vi "Func-엑셀 데이터를 그래프로 출력.vi"() -> ()   [LabVIEW 2015] (continued)
834.96\n834.98\n835\n835.01\n835.03\n835.04\n835.06\n835.08\n835.09\n835.11\n835.13\n835.14\n835.16\n835.18\n835.19\n835.21\n835.23\n835.24\n835.26\n835.28\n835.29\n835.31\n835.33\n835.34\n835.36\n835.38\n835.39\n835.41\n835.43\n835.44\n835.46\n835.48\n835.49\n835.51\n835.53\n835.54\n835.56\n835.58\n835.59\n835.61\n835.63\n835.64\n835.66\n835.68\n835.69\n835.71\n835.73\n835.74\n835.76\n835.78\n835.79\n835.81\n835.83\n835.84\n835.86\n835.88\n835.89\n835.91\n835.93\n835.94\n835.96\n835.98\n835.99\n836.01\n836.03\n836.04\n836.06\n836.08\n836.09\n836.11\n836.13\n836.14\n836.16\n836.18\n836.19\n836.21\n836.23\n836.24\n836.26\n836.28\n836.29\n836.31\n836.33\n836.34\n836.36\n836.38\n836.39\n836.41\n836.43\n836.44\n836.46\n836.48\n836.49\n836.51\n836.53\n836.54\n836.56\n836.58\n836.59\n836.61\n836.63\n836.64\n836.66\n836.68\n836.69\n836.71\n836.73\n836.74\n836.76\n836.78\n836.79\n836.81\n836.83\n836.84\n836.86\n836.88\n836.89\n836.91\n836.93\n836.94\n836.96\n836.98\n836.99\n837.01\n837.03\n837.04\n837.06\n837.08\n837.09\n837.11\n837.13\n837.14\n837.16\n837.18\n837.19\n837.21\n837.23\n837.24\n837.26\n837.28\n837.29\n837.31\n837.33\n837.34\n837.36\n837.38\n837.39\n837.41\n837.43\n837.44\n837.46\n837.48\n837.5\n837.51\n837.53\n837.54\n837.56\n837.58\n837.59\n837.61\n837.63\n837.64\n837.66\n837.68\n837.69\n837.71\n837.73\n837.75\n837.76\n837.78\n837.79\n837.81\n837.83\n837.85\n837.86\n837.88\n837.89\n837.91\n837.93\n837.94\n837.96\n837.98\n837.99\n838.01\n838.03\n838.04\n838.06\n838.08\n838.09\n838.11\n838.13\n838.14\n838.16\n838.18\n838.2\n838.21\n838.23\n838.24\n838.26\n838.28\n838.29\n838.31\n838.33\n838.34\n838.36\n838.38\n838.39\n838.41\n838.43\n838.44\n838.46\n838.48\n838.49\n838.51\n838.53\n838.54\n838.56\n838.58\n838.59\n838.61\n838.63\n838.65\n838.66\n838.68\n838.7\n838.71\n838.73\n838.74\n838.76\n838.78\n838.79\n838.81\n838.83\n838.84\n838.86\n838.88\n838.89\n838.91\n838.93\n838.94\n838.96\n838.98\n838.99\n839.01\n839.03\n839.05\n839.06\n839.08\n839.09\n839.11\n839.13\n839.14\n839.16\n839.18\n839.19\n839.21\n839.23\n839.24\n839.26\n839.28\n839.29\n839.31\n839.33\n839.34\n839.36\n839.38\n839.39\n839.41\n839.43\n839.44\n839.46\n839.48\n839.49\n839.51\n839.53\n839.54\n839.56\n839.58\n839.59\n839.61\n839.63\n839.64\n839.66\n839.68\n839.69\n839.71\n839.73\n839.74\n839.76\n839.78\n839.79\n839.81\n839.83\n839.84\n839.86\n839.88\n839.89\n839.91\n839.93\n839.94\n839.96\n839.98\n839.99\n840.01\n840.03\n840.04\n840.06\n840.08\n840.09\n840.11\n840.13\n840.15\n840.16\n840.18\n840.19\n840.21\n840.23\n840.25\n840.26\n840.28\n840.29\n840.31\n840.33\n840.34\n840.36\n840.38\n840.39\n840.41\n840.43\n840.44\n840.46\n840.48\n840.5\n840.51\n840.53\n840.54\n840.56\n840.58\n840.6\n840.61\n840.63\n840.64\n840.66\n840.68\n840.69\n840.71\n840.73\n840.74\n840.76\n840.78\n840.79\n840.81\n840.83\n840.85\n840.86\n840.88\n840.89\n840.91\n840.93\n840.95\n840.96\n840.98\n840.99\n841.01\n841.03\n841.04\n841.06\n841.08\n841.1\n841.11\n841.13\n841.14\n841.16\n841.18\n841.19\n841.21\n841.23\n841.24\n841.26\n841.28\n841.29\n841.31\n841.33\n841.34\n841.36\n841.38\n841.39\n841.41\n841.43\n841.45\n841.46\n841.48\n841.49\n841.51\n841.53\n841.54\n841.56\n841.58\n841.59\n841.61\n841.63\n841.64\n841.66\n841.68\n841.69\n841.71\n841.73\n841.74\n841.76\n841.78\n841.79\n841.81\n841.83\n841.84\n841.86\n841.88\n841.89\n841.91\n841.93\n841.94\n841.96\n841.98\n842\n842.01\n842.03\n842.04\n842.06\n842.08\n842.09\n842.11\n842.13\n842.14\n842.16\n842.18\n842.19\n842.21\n842.23\n842.24\n842.26\n842.28\n842.29\n842.31\n842.33\n842.34\n842.36\n842.38\n842.39\n842.41\n842.43\n842.44\n842.46\n842.48\n842.49\n842.51\n842.53\n842.54\n842.56\n842.58\n842.59\n842.61\n842.63\n842.64\n842.66\n842.68\n842.69\n842.71\n842.73\n842.74\n842.76\n842.78\n842.79\n842.81\n842.83\n842.84\n842.86\n842.88\n842.89\n842.91\n842.93\n842.94\n842.96\n842.98\n843\n843.01\n843.03\n843.04\n843.06\n843.08\n843.09\n843.11\n843.13\n843.14\n843.16\n843.18\n843.19\n843.21\n843.23\n843.25\n843.26\n843.28\n843.29\n843.31\n843.33\n843.34\n843.36\n843.38\n843.39\n843.41\n843.43\n843.44\n843.46\n843.48\n843.49\n843.51\n843.53\n843.54\n843.56\n843.58\n843.6\n843.61\n843.63\n843.64\n843.66\n843.68\n843.7\n843.71\n843.73\n843.74\n843.76\n843.78\n843.79\n843.81\n843.83\n843.85\n843.86\n843.88\n843.89\n843.91\n843.93\n843.95\n843.96\n843.98\n843.99\n844.01\n844.03\n844.04\n844.06\n844.08\n844.09\n844.11\n844.13\n844.14\n844.16\n844.18\n844.2\n844.21\n844.23\n844.24\n844.26\n844.28\n844.3\n844.31\n844.33\n844.34\n844.36\n844.38\n844.4\n844.41\n844.43\n844.44\n844.46\n844.48\n844.49\n844.51\n844.53\n844.55\n844.56\n844.58\n844.59\n844.61\n844.63\n844.64\n844.66\n844.68\n844.69\n844.71\n844.73\n844.74\n844.76\n844.78\n844.79\n844.81\n844.83\n844.84\n844.86\n844.88\n844.9\n844.91\n844.93\n844.94\n844.96\n844.98\n844.99\n845.01\n845.03\n845.04\n845.06\n845.08\n845.09\n845.11\n845.13\n845.14\n845.16\n845.18\n845.19\n845.21\n845.23\n845.24\n845.26\n845.28\n845.29\n845.31\n845.33\n845.34\n845.36\n845.38\n845.39\n845.41\n845.43\n845.44\n845.46\n845.48\n845.49\n845.51\n845.53\n845.54\n845.56\n845.58\n845.59\n845.61\n845.63\n845.64\n845.66\n845.68\n845.69\n845.71\n845.73\n845.74\n845.76\n845.78\n845.79\n845.81\n845.83\n845.84\n845.86\n845.88\n845.89\n845.91\n845.93\n845.94\n845.96\n845.98\n845.99\n846.01\n846.03\n846.04\n846.06\n846.08\n846.09\n846.11\n846.13\n846.14\n846.16\n846.18\n846.19\n846.21\n846.23\n846.24\n846.26\n846.28\n846.29\n846.31\n846.33\n846.35\n846.36\n846.38\n846.39\n846.41\n846.43\n846.44\n846.46\n846.48\n846.49\n846.51\n846.53\n846.54\n846.56\n846.58\n846.59\n846.61\n846.63\n846.64\n846.66\n846.68\n846.7\n846.71\n846.73\n846.74\n846.76\n846.78\n846.79\n846.81\n846.83\n846.84\n846.86\n846.88\n846.89\n846.91\n846.93\n846.95\n846.96\n846.98\n846.99\n847.01\n847.03\n847.05\n847.06\n847.08\n847.09\n847.11\n847.13\n847.14\n847.16\n847.18\n847.19\n847.21\n847.23\n847.24\n847.26\n847.28\n847.3\n847.31\n847.33\n847.34\n847.36\n847.38\n847.4\n847.41\n847.43\n847.44\n847.46\n847.48\n847.49\n847.51\n847.53\n847.55\n847.56\n847.58\n847.59\n847.61\n847.63\n847.64\n847.66\n847.68\n847.69\n847.71\n847.73\n847.75\n847.76\n847.78\n847.79\n847.81\n847.83\n847.84\n847.86\n847.88\n847.9\n847.91\n847.93\n847.94\n847.96\n847.98\n848\n848.01\n848.03\n848.04\n848.06\n848.08\n848.09\n848.11\n848.13\n848.15\n848.16\n848.18\n848.19\n848.21\n848.23\n848.24\n848.26\n848.28\n848.29\n848.31\n848.33\n848.34\n848.36\n848.38\n848.39\n848.41\n848.43\n848.44\n848.46\n848.48\n848.49\n848.51\n848.53\n848.54\n848.56\n848.58\n848.59\n848.61\n848.63\n848.64\n848.66\n848.68\n848.69\n848.71\n848.73\n848.74\n848.76\n848.78\n848.79\n848.81\n848.83\n848.84\n848.86\n848.88\n848.89\n848.91\n848.93\n848.94\n848.96\n848.98\n848.99\n849.01\n849.03\n849.04\n849.06\n849.08\n849.09\n849.11\n849.13\n849.14\n849.16\n849.18\n849.19\n849.21\n849.23\n849.24\n849.26\n849.28\n849.29\n849.31\n849.33\n849.34\n849.36\n849.38\n849.39\n849.41\n849.43\n849.45\n849.46\n849.48\n849.49\n849.51\n849.53\n849.54\n849.56\n849.58\n849.59\n849.61\n849.63\n849.64\n849.66\n849.68\n849.7\n849.71\n849.73\n849.74\n849.76\n849.78\n849.8\n849.81\n849.83\n849.84\n849.86\n849.88\n849.89\n849.91\n849.93\n849.94\n849.96\n849.98\n849.99\n850.01\n850.03\n850.05\n850.06\n850.08\n850.09\n850.11\n850.13\n850.15\n850.16\n850.18\n850.19\n850.21\n850.23\n850.24\n850.26\n850.28\n850.29\n850.31\n850.33\n850.34\n850.36\n850.38\n850.39\n850.41\n850.43\n850.44\n850.46\n850.48\n850.5\n850.51\n850.53\n850.54\n850.56\n850.58\n850.6\n850.61\n850.63\n850.64\n850.66\n850.68\n850.69\n850.71\n850.73\n850.74\n850.76\n850.78\n850.79\n850.81\n850.83\n850.85\n850.86\n850.88\n850.89\n850.91\n850.93\n850.94\n850.96\n850.98\n850.99\n851.01\n851.03\n851.04\n851.06\n851.08\n851.1\n851.11\n851.13\n851.14\n851.16\n851.18\n851.19\n851.21\n851.23\n851.24\n851.26\n851.28\n851.29\n851.31\n851.33\n851.34\n851.36\n851.38\n851.39\n851.41\n851.43\n851.44\n851.46\n851.48\n851.49\n851.51\n851.53\n851.54\n851.56\n851.58\n851.59\n851.61\n851.63\n851.64\n851.66\n851.68\n851.69\n851.71\n851.73\n851.74\n851.76\n851.78\n851.79\n851.81\n851.83\n851.84\n851.86\n851.88\n851.89\n851.91\n851.93\n851.94\n851.96\n851.98\n851.99\n852.01\n852.03\n852.04\n852.06\n852.08\n852.09\n852.11\n852.13\n852.14\n852.16\n852.18\n852.19\n852.21\n852.23\n852.24\n852.26\n852.28\n852.29\n852.31\n852.33\n852.34\n852.36\n852.38\n852.39\n852.41\n852.43\n852.44\n852.46\n852.48\n852.49\n852.51\n852.53\n852.54\n852.56\n852.58\n852.59\n852.61\n852.63\n852.64\n852.66\n852.68\n852.69\n852.71\n852.73\n852.74\n852.76\n852.78\n852.8\n852.81\n852.83\n852.84\n852.86\n852.88\n852.9\n852.91\n852.93\n852.94\n852.96\n852.98\n852.99\n853.01\n853.03\n853.04\n853.06\n853.08\n853.09\n853.11\n853.13\n853.15\n853.16\n853.18\n853.19\n853.21\n853.23\n853.25\n853.26\n853.28\n853.29\n853.31\n853.33\n853.34\n853.36\n853.38\n853.39\n853.41\n853.43\n853.44\n853.46\n853.48\n853.5\n853.51\n853.53\n853.54\n853.56\n853.58\n853.59\n853.61\n853.63\n853.64\n853.66\n853.68\n853.7\n853.71\n853.73\n853.74\n853.76\n853.78\n853.79\n853.81\n853.83\n853.84\n853.86\n853.88\n853.89\n853.91\n853.93\n853.94\n853.96\n853.98\n853.99\n854.01\n854.03\n854.04\n854.06\n854.08\n854.1\n854.11\n854.13\n854.14\n854.16\n854.18\n854.2\n854.21\n854.23\n854.24\n854.26\n854.28\n854.29\n854.31\n854.33\n854.34\n854.36\n854.38\n854.39\n854.41\n854.43\n854.44\n854.46\n854.48\n854.49\n854.51\n854.53\n854.54\n854.56\n854.58\n854.59\n854.61\n854.63\n854.64\n854.66\n854.68\n854.69\n854.71\n854.73\n854.74\n854.76\n854.78\n854.79\n854.81\n854.83\n854.84\n854.86\n854.88\n854.89\n854.91\n854.93\n854.94\n854.96\n854.98\n854.99\n855.01\n855.03\n855.04\n855.06\n855.08\n855.09\n855.11\n855.13\n855.14\n855.16\n855.18\n855.19\n855.21\n855.23\n855.24\n855.26\n855.28\n855.29\n855.31\n855.33\n855.34\n855.36\n855.38\n855.39\n855.41\n855.43\n855.44\n855.46\n855.48\n855.49\n855.51\n855.53\n855.55\n855.56\n855.58\n855.59\n855.61\n855.63\n855.64\n855.66\n855.68\n855.69\n855.71\n855.73\n855.74\n855.76\n855.78\n855.79\n855.81\n855.83\n855.84\n855.86\n855.88\n855.9\n855.91\n855.93\n855.94\n855.96\n855.98\n856\n856.01\n856.03\n856.04\n856.06\n856.08\n856.09\n856.11\n856.13\n856.15\n856.16\n856.18\n856.19\n856.21\n856.23\n856.25\n856.26\n856.28\n856.29\n856.31\n856.33\n856.35\n856.36\n856.38\n856.39\n856.41\n856.43\n856.44\n856.46\n856.48\n856.49\n856.51\n856.53\n856.54\n856.56\n856.58\n856.6\n856.61\n856.63\n856.64\n856.66\n856.68\n856.69\n856.71\n856.73\n856.74\n856.76\n856.78\n856.79\n856.81\n856.83\n856.84\n856.86\n856.88\n856.89\n856.91\n856.93\n856.94\n856.96\n856.98\n856.99\n857.01\n857.03\n857.05\n857.06\n857.08\n857.1\n857.11\n857.13\n857.14\n857.16\n857.18\n857.19\n857.21\n857.23\n857.24\n857.26\n857.28\n857.3\n857.31\n857.33\n857.34\n857.36\n857.38\n857.39\n857.41\n857.43\n857.44\n857.46\n857.48\n857.49\n857.51\n857.53\n857.54\n857.56\n857.58\n857.59\n857.61\n857.63\n857.64\n857.66\n857.68\n857.69\n857.71\n857.73\n857.74\n857.76\n857.78\n857.79\n857.81\n857.83\n857.84\n857.86\n857.88\n857.89\n857.91\n857.93\n857.94\n857.96\n857.98\n857.99\n858.01\n858.03\n858.04\n858.06\n858.08\n858.09\n858.11\n858.13\n858.14\n858.16\n858.18\n858.19\n858.21\n858.23\n858.24\n858.26\n858.28\n858.29\n858.31\n858.33\n858.34\n858.36\n858.38\n858.39\n858.41\n858.43\n858.44\n858.46\n858.48\n858.49\n858.51\n858.53\n858.54\n858.56\n858.58\n858.59\n858.61\n858.63\n858.64\n858.66\n858.68\n858.69\n858.71\n858.73\n858.74\n858.76\n858.78\n858.79\n858.81\n858.83\n858.84\n858.86\n858.88\n858.89\n858.91\n858.93\n858.94\n858.96\n858.98\n859\n859.01\n859.03\n859.04\n859.06\n859.08\n859.09\n859.11\n859.13\n859.14\n859.16\n859.18\n859.19\n859.21\n859.23\n859.25\n859.26\n859.28\n859.29\n859.31\n859.33\n859.35\n859.36\n859.38\n859.39\n859.41\n859.43\n859.45\n859.46\n859.48\n859.49\n859.51\n859.53\n859.54\n859.56\n859.58\n859.59\n859.61\n859.63\n859.64\n859.66\n859.68\n859.69\n859.71\n859.73\n859.74\n859.76\n859.78\n859.79\n859.81\n859.83\n859.84\n859.86\n859.88\n859.89\n859.91\n859.93\n859.94\n859.96\n859.98\n859.99\n860.01\n860.03\n860.04\n860.06\n860.08\n860.09\n860.11\n860.13\n860.14\n860.16\n860.18\n860.19\n860.21\n860.23\n860.24\n860.26\n860.28\n860.3\n860.31\n860.33\n860.34\n860.36\n860.38\n860.39\n860.41\n860.43\n860.44\n860.46\n860.48\n860.49\n860.51\n860.53\n860.54\n860.56\n860.58\n860.59\n860.61\n860.63\n860.64\n860.66\n860.68\n860.69\n860.71\n860.73\n860.74\n860.76\n860.78\n860.79\n860.81\n860.83\n860.84\n860.86\n860.88\n860.89\n860.91\n860.93\n860.94\n860.96\n860.98\n860.99\n861.01\n861.03\n861.04\n861.06\n861.08\n861.09\n861.11\n861.13\n861.14\n861.16\n861.18\n861.19\n861.21\n861.23\n861.24\n861.26\n861.28\n861.29\n861.31\n861.33\n861.34\n861.36\n861.38\n861.39\n861.41\n861.43\n861.44\n861.46\n861.48\n861.49\n861.51\n861.53\n861.54\n861.56\n861.58\n861.59\n861.61\n861.63\n861.64\n861.66\n861.68\n861.69\n861.71\n861.73\n861.74\n861.76\n861.78\n861.79\n861.81\n861.83\n861.84\n861.86\n861.88\n861.89\n861.91\n861.93\n861.94\n861.96\n861.98\n862\n862.01\n862.03\n862.04\n862.06\n862.08\n862.1\n862.11\n862.13\n862.14\n862.16\n862.18\n862.19\n862.21\n862.23\n862.24\n862.26\n862.28\n862.29\n862.31\n862.33\n862.35\n862.36\n862.38\n862.39\n862.41\n862.43\n862.45\n862.46\n862.48\n862.49\n862.51\n862.53\n862.54\n862.56\n862.58\n862.6\n862.61\n862.63\n862.64\n862.66\n862.68\n862.7\n862.71\n862.73\n862.74\n862.76\n862.78\n862.79\n862.81\n862.83\n862.84\n862.86\n862.88\n862.89\n862.91\n862.93\n862.94\n862.96\n862.98\n862.99\n863.01\n863.03\n863.04\n863.06\n863.08\n863.09\n863.11\n863.13\n863.14\n863.16\n863.18\n863.19\n863.21\n863.23\n863.24\n863.26\n863.28\n863.29\n863.31\n863.33\n863.34\n863.36\n863.38\n863.39\n863.41\n863.43\n863.44\n863.46\n863.48\n863.49\n863.51\n863.53\n863.54\n863.56\n863.58\n863.59\n863.61\n863.63\n863.64\n863.66\n863.68\n863.69\n863.71\n863.73\n863.74\n863.76\n863.78\n863.79\n863.81\n863.83\n863.84\n863.86\n863.88\n863.89\n863.91\n863.93\n863.94\n863.96\n863.98\n863.99\n864.01\n864.03\n864.04\n864.06\n864.08\n864.09\n864.11\n864.13\n864.14\n864.16\n864.18\n864.19\n864.21\n864.23\n864.24\n864.26\n864.28\n864.29\n864.31\n864.33\n864.34\n864.36\n864.38\n864.39\n864.41\n864.43\n864.44\n864.46\n864.48\n864.49\n864.51\n864.53\n864.54\n864.56\n864.58\n864.59\n864.61\n864.63\n864.64\n864.66\n864.68\n864.69\n864.71\n864.73\n864.75\n864.76\n864.78\n864.79\n864.81\n864.83\n864.84\n864.86\n864.88\n864.89\n864.91\n864.93\n864.94\n864.96\n864.98\n864.99\n865.01\n865.03\n865.04\n865.06\n865.08\n865.1\n865.11\n865.13\n865.14\n865.16\n865.18\n865.2\n865.21\n865.23\n865.24\n865.26\n865.28\n865.29\n865.31\n865.33\n865.35\n865.36\n865.38\n865.39\n865.41\n865.43\n865.45\n865.46\n865.48\n865.49\n865.51\n865.53\n865.55\n865.56\n865.58\n865.59\n865.61\n865.63\n865.64\n865.66\n865.68\n865.7\n865.71\n865.73\n865.74\n865.76\n865.78\n865.8\n865.81\n865.83\n865.84\n865.86\n865.88\n865.9\n865.91\n865.93\n865.94\n865.96\n865.98\n865.99\n866.01\n866.03\n866.04\n866.06\n866.08\n866.09\n866.11\n866.13\n866.15\n866.16\n866.18\n866.19\n866.21\n866.23\n866.24\n866.26\n866.28\n866.29\n866.31\n866.33\n866.34\n866.36\n866.38\n866.39\n866.41\n866.43\n866.44\n866.46\n866.48\n866.49\n866.51\n866.53\n866.54\n866.56\n866.58\n866.59\n866.61\n866.63\n866.65\n866.66\n866.68\n866.69\n866.71\n866.73\n866.74\n866.76\n866.78\n866.79\n866.81\n866.83\n866.84\n866.86\n866.88\n866.89\n866.91\n866.93\n866.94\n866.96\n866.98\n866.99\n867.01\n867.03\n867.04\n867.06\n867.08\n867.09\n867.11\n867.13\n867.14\n867.16\n867.18\n867.19\n867.21\n867.23\n867.24\n867.26\n867.28\n867.29\n867.31\n867.33\n867.34\n867.36\n867.38\n867.39\n867.41\n867.43\n867.44\n867.46\n867.48\n867.49\n867.51\n867.53\n867.54\n867.56\n867.58\n867.59\n867.61\n867.63\n867.64\n867.66\n867.68\n867.69\n867.71\n867.73\n867.74\n867.76\n867.78\n867.79\n867.81\n867.83\n867.84\n867.86\n867.88\n867.89\n867.91\n867.93\n867.94\n867.96\n867.98\n867.99\n868.01\n868.03\n868.04\n868.06\n868.08\n868.09\n868.11\n868.13\n868.14\n868.16\n868.18\n868.2\n868.21\n868.23\n868.24\n868.26\n868.28\n868.29\n868.31\n868.33\n868.34\n868.36\n868.38\n868.39\n868.41\n868.43\n868.45\n868.46\n868.48\n868.49\n868.51\n868.53\n868.55\n868.56\n868.58\n868.59\n868.61\n868.63\n868.64\n868.66\n868.68\n868.69\n868.71\n868.73\n868.74\n868.76\n868.78\n868.8\n868.81\n868.83\n868.84\n868.86\n868.88\n868.9\n868.91\n868.93\n868.94\n868.96\n868.98\n869\n869.01\n869.03\n869.04\n869.06\n869.08\n869.09\n869.11\n869.13\n869.14\n869.16\n869.18\n869.19\n869.21\n869.23\n869.24\n869.26\n886.44\n886.61\n886.77\n886.94\n887.11\n887.27\n887.44\n887.61\n887.77\n887.94\n888.11\n888.27\n888.44\n888.61\n888.77\n888.94\n889.11\n889.27\n889.44\n889.61\n889.77\n889.94\n890.11\n890.27\n890.44\n890.61\n890.77\n890.94\n891.11\n891.27\n891.44\n891.61\n891.77\n891.94\n892.11\n892.27\n892.44\n892.61\n892.77\n892.94\n893.11\n893.27\n893.44\n893.61\n893.77\n893.94\n894.11\n894.28\n894.45\n894.61\n894.78\n894.95\n895.11\n895.28\n895.45\n895.61\n895.78\n895.95\n896.11\n896.28\n896.45\n896.61\n896.78\n896.95\n897.11\n897.28\n897.45\n897.61\n897.78\n897.95\n898.11\n898.28\n898.45\n898.61\n898.78\n898.95\n899.11\n899.28\n899.45\n899.61\n899.79\n899.96\n900.12\n900.29\n900.46\n900.62\n900.79\n900.96\n901.12\n901.29\n901.46\n901.62\n901.79\n901.96\n902.12\n902.29\n902.46\n902.62\n902.79\n902.96\n903.12\n903.29\n903.46\n903.62\n903.79\n903.96\n904.12\n904.29\n904.46\n904.62\n904.79\n904.96\n905.12\n905.29\n905.46\n905.62\n905.79\n905.96\n906.12\n906.29\n906.46\n906.62\n906.79\n906.96\n907.12\n907.29\n907.46\n907.62\n907.79\n907.96\n908.12\n908.29\n908.46\n908.62\n908.79\n908.96\n909.12\n909.29\n909.46\n909.62\n909.79\n909.96\n910.12\n910.29\n910.46\n910.62\n910.79\n910.97\n911.13\n911.3\n911.46\n911.63\n911.8\n911.96\n912.13\n912.3\n912.46\n912.63\n912.8\n912.96\n913.13\n913.3\n913.46\n913.63\n913.8\n913.97\n914.13\n914.3\n914.46\n914.63\n914.8\n914.96\n915.13\n915.3\n915.46\n915.64\n915.81\n915.97\n916.14\n916.31\n916.47\n916.64\n916.81\n916.97\n917.14\n917.31\n917.47\n917.64\n917.81\n917.97\n918.14\n918.31\n918.47\n918.64\n918.81\n918.97\n919.14\n919.31\n919.47\n919.64\n919.81\n919.97\n920.14\n920.31\n920.47\n920.64\n920.81\n920.97\n921.14\n921.31\n921.47\n921.64\n921.81\n921.97\n922.14\n922.31\n922.47\n922.65\n922.82\n922.98\n923.16\n923.32\n923.49\n923.66\n923.82\n923.99\n924.16\n924.32\n924.49\n924.66\n924.83\n925\n925.16\n925.33\n925.5\n925.66\n925.83\n926\n926.17\n926.33\n926.49\n926.49\n926.51\n926.53\n926.54\n926.56\n926.58\n926.59\n926.61\n926.63\n926.64\n926.66\n926.68\n926.69\n926.71\n926.73\n926.74\n926.76\n926.78\n926.79\n926.81\n926.83\n926.85\n926.86\n926.88\n926.89\n926.91\n926.93\n926.94\n926.96\n926.98\n926.99\n927.01\n927.03\n927.04\n927.06\n927.08\n927.09\n927.11\n927.13\n927.15\n927.16\n927.18\n927.19\n927.21\n927.23\n927.24\n927.26\n927.28\n927.29\n927.31\n927.33\n927.34\n927.36\n927.38\n927.39\n927.41\n927.43\n927.44\n927.46\n927.48\n927.49\n927.51\n927.53\n927.54\n927.56\n927.58\n927.59\n927.61\n927.63\n927.64\n927.66\n927.68\n927.69\n927.71\n927.73\n927.74\n927.76\n927.78\n927.79\n927.81\n927.83\n927.84\n927.86\n927.88\n927.89\n927.91\n927.93\n927.94\n927.96\n927.98\n927.99\n928.01\n928.03\n928.04\n928.06\n928.08\n928.09\n928.11\n928.13\n928.14\n928.16\n928.18\n928.19\n928.21\n928.23\n928.24\n928.26\n928.28\n928.29\n928.31\n928.33\n928.34\n928.36\n928.38\n928.39\n928.41\n928.43\n928.44\n928.46\n928.48\n928.49\n928.51\n928.53\n928.54\n928.56\n928.58\n928.59\n928.61\n928.63\n928.65\n928.66\n928.68\n928.69\n928.71\n928.73\n928.74\n928.76\n928.78\n928.79\n928.81\n928.83\n928.84\n928.86\n928.88\n928.9\n928.91\n928.93\n928.94\n928.96\n928.98\n929\n929.01\n929.03\n929.04\n929.06\n929.08\n929.1\n929.11\n929.13\n929.14\n929.16\n929.18\n929.19\n929.21\n929.23\n929.25\n929.26\n929.28\n929.29\n929.31\n929.33\n929.35\n929.36\n929.38\n929.39\n929.41\n929.43\n929.45\n929.46\n929.48\n929.49\n929.51\n929.53\n929.54\n929.56\n929.58\n929.59\n929.61\n929.63\n929.64\n929.66\n929.68\n929.69\n929.71\n929.73\n929.74\n929.76\n929.78\n929.79\n929.81\n929.83\n929.84\n929.86\n929.88\n929.89\n929.91\n929.93\n929.94\n929.96\n929.98\n929.99\n
